vi "FindProjectPath.vi"(6 "BuildSpecs? (F)":bool, 8 "error in (no error)":errorcluster, 11 "Library/Class Name":string) -> (0 "error out":errorcluster, 2 "Found?":bool, 3 "Project Path":path)   [LabVIEW 2019, in "DepsWatch.lvlib"]
uses:
  DepsWatch.lvlib
  <vilib>/SLL Toolkit/SLL String/SLL String.lvlib
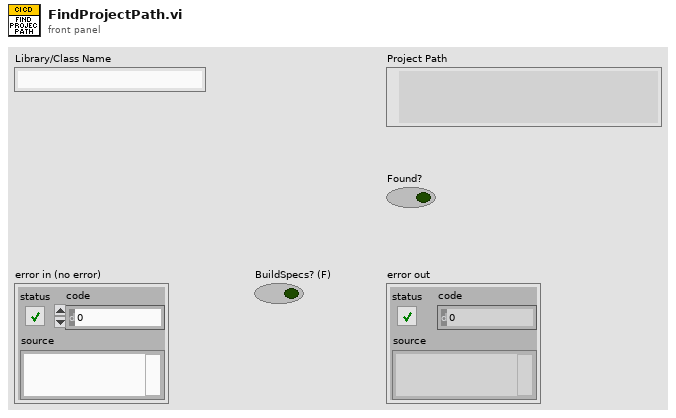
[diagram p1: front panel]
types:
  T1 = typedef "DepsWatch.lvlib/CICDPathConfigs.ctl" = cluster{"GlobalIncludePaths":path[], "GlobalExcludePaths":path[], "BuildSpecsIncludePaths":path[], "ActualDepsIncludePaths":path[], "WorkspacePath":path, "SourceFolderPaths":path[], "ChangedFilesLogpaths":map{string, path}}
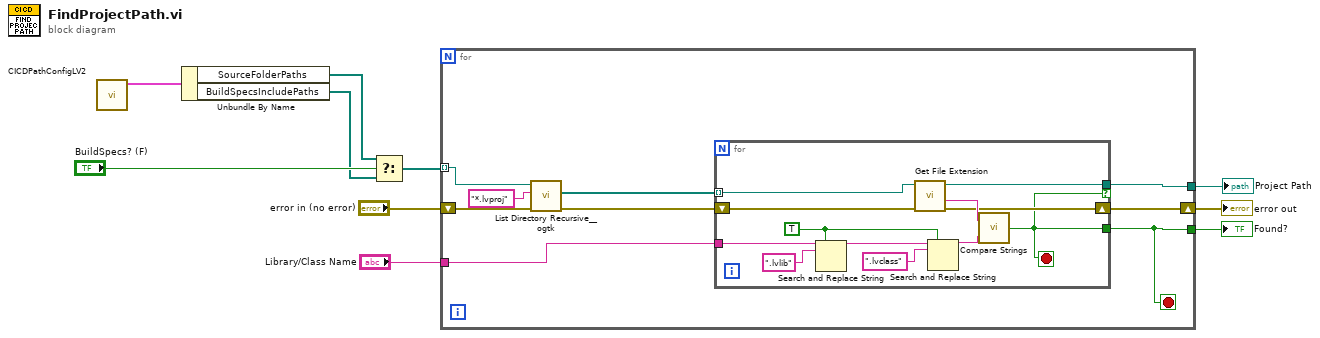
[diagram p0: block diagram]
diagram:
  n1 = call "CICDPathConfigLV2.vi"() -> ("CICD Path Config Out"=w5:T1)  [unwired: 11 in]
  n2 = Unbundle By Name(w5) -> ("SourceFolderPaths"=w2:path[], "BuildSpecsIncludePaths"=w3:path[])
  n3 = Select(t=w2, s="BuildSpecs? (F)", f=w3) -> (s? t:f=w1:path[])
  n4 = for {
    tunnel: [w18] -> w9
    tunnel: [w11] -> w8
    tunnel: "Library/Class Name" -> [w16]
    shift-right: [w13] -> w6
    shift-left: "error in (no error)" -> [w19]
    tunnel: w1 -> [w12] mode=indexing
    stop <- w11 stop-if-true
    n5 = call <userlib>:"List Directory Recursive__ogtk.vi"("error in (no error)"=w19, "pattern"="*.lvproj", "Path"=w12) -> ("error out"=w17:errorcluster, "file paths"=w15:path[])  [unwired: 5 in, 2 out]
    n6 = for {
      tunnel: w15 -> [w30] mode=indexing
      tunnel: w16 -> [w21]
      shift-right: [w26] -> w13
      shift-left: w17 -> [w31]
      tunnel: [w25] -> w18 if=w24
      tunnel: [w24] -> w11
      stop <- w24 stop-if-true
      w20 = TRUE ("replace all? (F)")
      n7 = Search and Replace String(replace all?=w20, input string=w21, search string=".lvlib") -> (result string=w22:string)  [unwired: 5 in, 3 out]
      n8 = call <vilib>:"Get File Extension.vi"("error in (no error)"=w31, "file"=w30) -> ("error out"=w26:errorcluster, "filename without extension"=w28:string, "dup file"=w25:path)  [unwired: 5 in, 2 out]
      n9 = Search and Replace String(replace all?=w20, input string=w22, search string=".lvclass") -> (result string=w27:string)  [unwired: 5 in, 3 out]
      n10 = call <vilib>:"Compare Strings.vi"("y"=w27, "x"=w28) -> ("Equal?"=w24:bool)
    }
  }
  "Project Path" <- w9
  "Found?" <- w8
  "error out" <- w6
